vi "Initialize.vi"(8 "error in":errorcluster, 10 "DataGridView":refnum<k24>(container), 11 "DataGrid in":refnum<class "DataGridView.lvclass">) -> (0 "error out":errorcluster, 3 "DataGrid out":refnum<class "DataGridView.lvclass">)   [LabVIEW 2013, in "DataGrid.lvlib" / "DataGridView.lvclass"]
doc: "Sets all the initial default values of various properties to make a datagrid more user friendly. These can be modified thorugh the class properties, they are simple all set together in this default initialization."
uses:
  DataGridView.lvclass
  DataGridView.lvclass/DataGridView.ctl
  Properties/Write AllowUserToResizeRows.vi
  Properties/Write AllowUserToOrderColumns.vi
  Properties/Write AllowUserToResizeColumns.vi
  Properties/Write RowHeadersVisible.vi
  Properties/Write AllowUserToAddRows.vi
  Properties/Write AutoSizeColumnsMode.vi
  Properties/Write AutoSizeRowsMode.vi
  Properties/Write DefaultCellBGKColor.vi
  Properties/Write DefaultAlternateCellBGKColor.vi
  Properties/Write SelectionMode.vi
  System.Windows.Forms
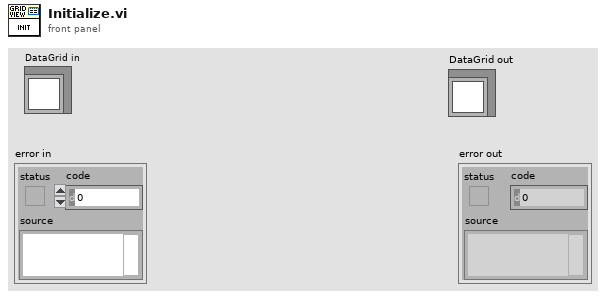
[diagram p1: front panel]
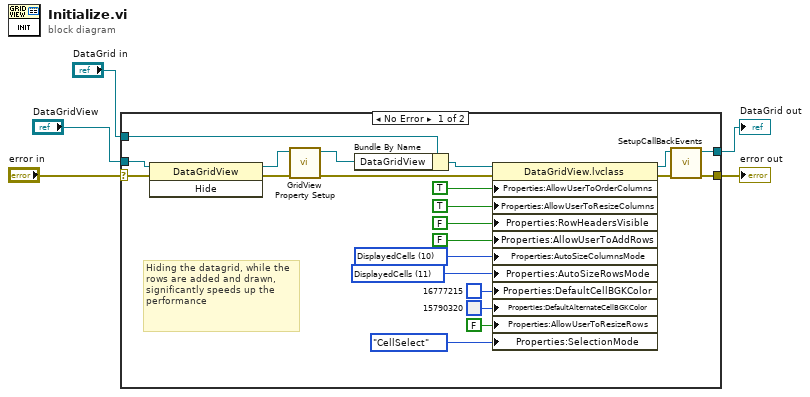
[diagram p0: block diagram]
diagram:
  n1 = case shown="No Error" "error in" {
    selector: "error in" -> [w24 w29]
    tunnel: [w26 w29] -> w4
    tunnel: [w25 w28] -> w2
    tunnel: "DataGrid in" -> [w27 w28]
    tunnel: "DataGridView" -> [w23 _]
    frame No Error {
      w14 = 11 items=["None"=0, "AllHeaders"=5, "AllCellsExceptHeaders"=6, "AllCells"=7, "DisplayedHeaders"=9, "DisplayedCellsExceptHeaders"=10, "DisplayedCells"=11] ("AutoSizeRowsMode")
      w15 = 10 items=["None"=1, "ColumnHeader"=2, "AllCellsExceptHeader"=4, "AllCells"=6, "DisplayedCellsExceptHeader"=8, "DisplayedCells"=10, "Fill"=16] ("AutoSizeColumnsMode")
      # "Hiding the datagrid, while the rows are added and drawn, significantly speeds up the performance"
      n2 = invoke class="DataGridView" method="Hide"(reference=w23, error in=w24) -> (reference out=w20:refnum<k24>, error out=w22:errorcluster)  [unwired: 1 in, 1 out]
      n3 = call "GridView Property Setup.vi"("error in (no error)"=w22, ".NET Refnum in"=w20) -> ("error out"=w21:errorcluster, ".NET Refnum out"=w19:refnum<k24>)  [unwired: 8 in]
      n4 = Bundle By Name(cluster=w27, "DataGridView"=w19) -> (w16:refnum<class "DataGridView.lvclass">)
      n5 = property class="DataGridView.lvclass"(reference=w16, error in=w21, "Properties:AllowUserToOrderColumns"=TRUE ("AllowUserToOrderColumns"), "Properties:AllowUserToResizeColumns"=TRUE ("AllowUserToResizeColumns"), "Properties:RowHeadersVisible"=FALSE ("RowHeadersVisible"), "Properties:AllowUserToAddRows"=FALSE ("AllowUserToAddRows"), "Properties:AutoSizeColumnsMode"=w15, "Properties:AutoSizeRowsMode"=w14, "Properties:DefaultCellBGKColor"=u32 16777215, "Properties:DefaultAlternateCellBGKColor"=u32 15790320, "Properties:AllowUserToResizeRows"=FALSE ("AllowUserToResizeRows"), "Properties:SelectionMode"=enum16{"CellSelect", "FullRowSelect"}."CellSelect" ("SelectionMode")) -> (reference out=w10:refnum<class "DataGridView.lvclass">, error out=w9:errorcluster)
      n6 = call "SetupCallBackEvents.vi"("error in (no error)"=w9, "DataGridView in"=w10) -> ("error out"=w26:errorcluster, "DataGridView out"=w25:refnum<class "DataGridView.lvclass">)  [unwired: 8 in]
    }
    frame Error {
    }
  }
  "error out" <- w4
  "DataGrid out" <- w2
